vi "Tarea_Progra.vi"() -> ()   [LabVIEW 2011]
panel:
  out "Nivel Maximo":bool
  out "Nivel Medio":bool
  out "Foco":bool
  in  "stop":bool
  in  "On/Off":bool
  in  "Knob":i32(knob) scale=0.0..4.0
  out "Tank":i32(slide) scale=0.0..80.0
  # "El Programa debera funcionar hasta que se presione el boton de detener\nEl Led debera de encender en la pc y en la proto usando el pulsador\nLos Niveles Maximos y Minimos deberan de encender en la Pc y en la Proto\nEl tanque se debera llenar usando el Knob que es una señal analogica. 1 equivale a 20\nMedio es 50 y Maximo es 80"
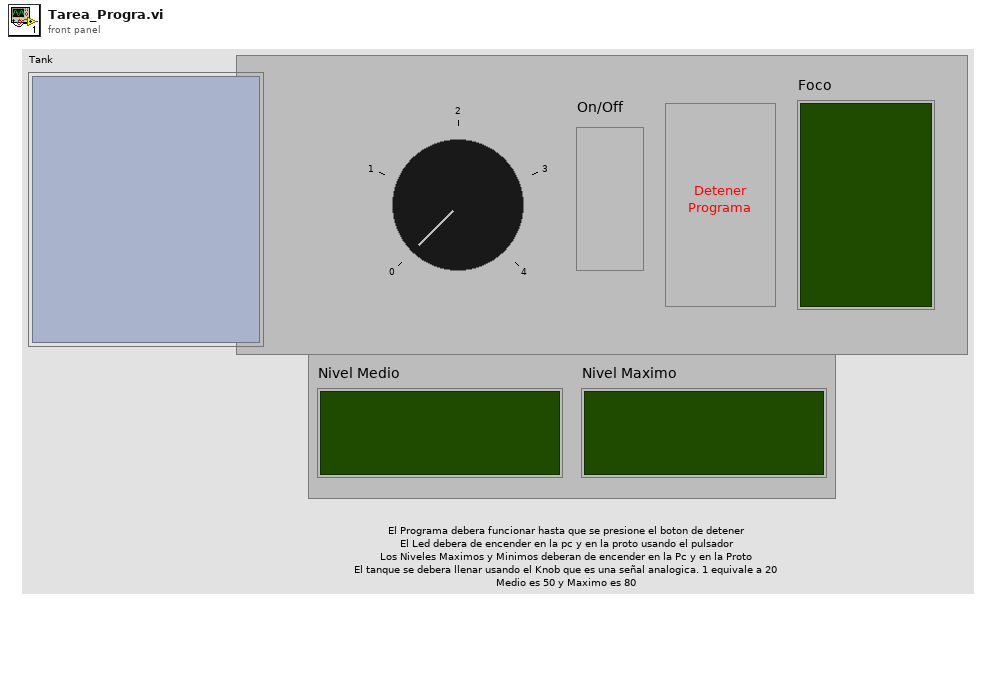
[diagram p1: front panel]
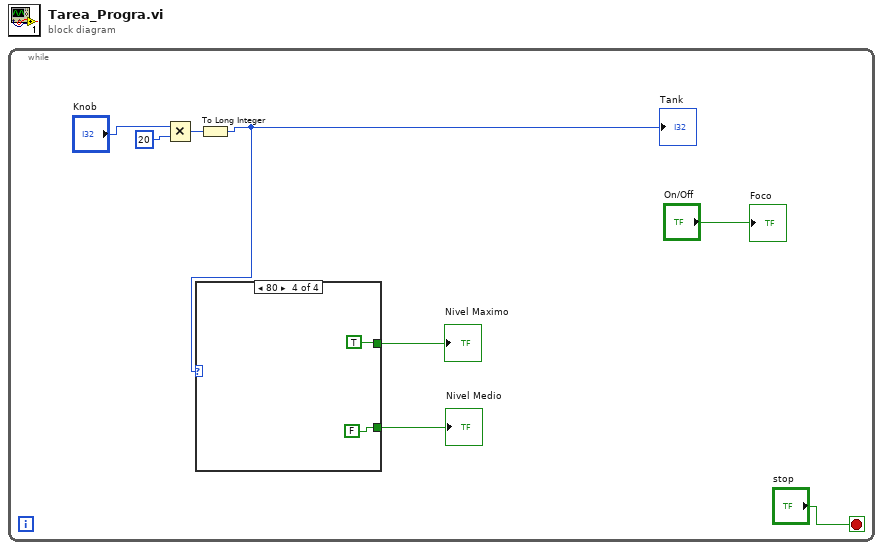
[diagram p0: block diagram]
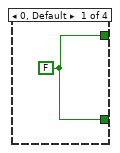
[diagram p2: hidden frame]
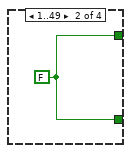
[diagram p3: hidden frame]
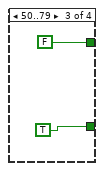
[diagram p4: hidden frame]
diagram:
  n1 = while {
    stop <- "stop" stop-if-true
    n2 = Multiply(x="Knob", y=20) -> (x*y=w4:i32)
    n3 = To Long Integer(number=w4) -> (32bit integer=w3:i32)
    "Tank" <- w3
    n4 = case shown="80" w3 {
      tunnel: [w9 w10 FALSE TRUE] -> w2
      tunnel: [w9 w10 TRUE FALSE] -> w1
      frame 0, Default {
        w9 = FALSE
      }
      frame 1..49 {
        w10 = FALSE
      }
      frame 50..79 {
      }
      frame 80 {
      }
    }
    "Nivel Maximo" <- w2
    "Nivel Medio" <- w1
    "Foco" <- "On/Off"
  }
